vi "nivision_about.vi"(8 "error in (no error)":errorcluster) -> (0 "error out":errorcluster)   [LabVIEW 2017]
uses:
  593b216a-fc24-450b-a2a5-084fb9140769.vi
panel:
  # "Designed And Developed By : NIVISION Pune"
  # "https://www.nivision.co.in"
  # "Contact :-9325640282"
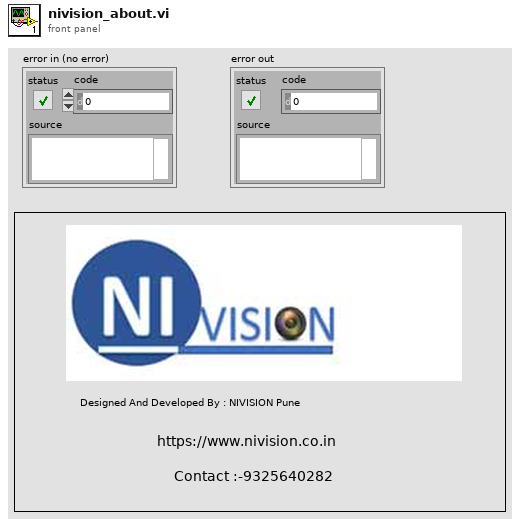
[diagram p1: front panel]
types:
  T1 = enum32{"invalid app kind", "Development System", "Run Time System", "Student Edition", "Embedded LabVIEW", "Evaluation", "Custom"}
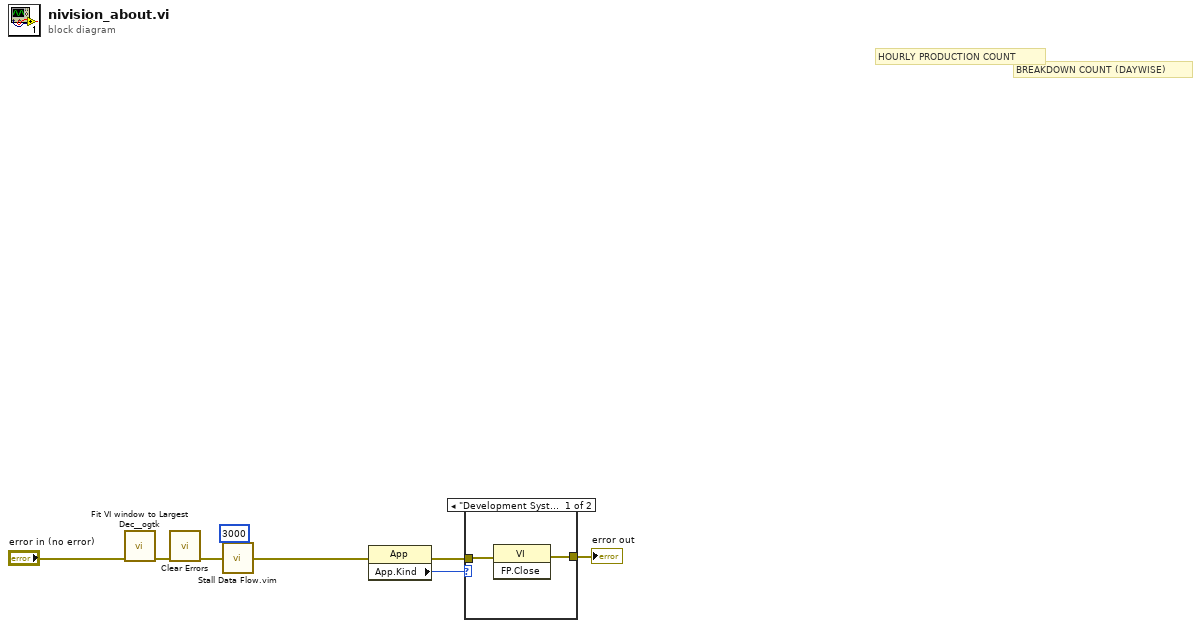
[diagram p0: block diagram]
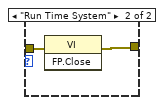
[diagram p2: hidden frame]
diagram:
  # "HOURLY PRODUCTION COUNT"
  # "BREAKDOWN COUNT (DAYWISE)"
  n1 = call <userlib>:"Fit VI window to Largest Dec__ogtk.vi"("error in (no error)"="error in (no error)") -> ("error out"=w2:errorcluster)  [unwired: 5 in, 1 out]
  n2 = call <vilib>:"Clear Errors.vi"("error in (no error)"=w2) -> ("error out"=w1:errorcluster)  [unwired: 5 in, 1 out]
  n3 = call "Stall Data Flow.vim"("value in"=w1, "milliseconds to wait"=u32 3000) -> ("value out"=w5:errorcluster)  [unwired: 1 out]
  n4 = property class="App"(error in=w5) -> (error out=w8:errorcluster, "App.Kind"=w7:T1)  [unwired: 1 in, 1 out]
  n5 = case shown="\"Development System\", Default" w7 {
    tunnel: w8 -> [w10 w12]
    tunnel: [w9 w11] -> w6
    frame "Development System", Default {
      n6 = invoke class="VI" method="FP.Close"(error in=w10) -> (error out=w9:errorcluster)  [unwired: 2 in, 2 out]
    }
    frame "Run Time System" {
      n7 = invoke class="VI" method="FP.Close"(error in=w12) -> (error out=w11:errorcluster)  [unwired: 2 in, 2 out]
    }
  }
  "error out" <- w6
